vi "Do.vi"(8 "error in (no error)":errorcluster, 9 "Events":refnum<class "Events.lvclass">, 10 "Message Loop Data in":T1, 11 "IRegister in":refnum<class "IRegister.lvclass">) -> (0 "error out":errorcluster, 1 "Write request":T10, 2 "Message Loop Data out":T1, 3 "IRegister out":refnum<class "IRegister.lvclass">)   [LabVIEW 2020, in "wamplv.lvlib" / "IRegister.lvclass"]
uses:
  IRegister.lvclass
  WAMP Client/API/TypeDefs/WAMP error (JSON).ctl
  wamplv.lvlib
  WAMP Client/API/TypeDefs/Combined error.ctl
  WAMP Client/Private/TypeDef/Success or error (JSON).ctl
  WAMP Client/Private/TypeDef/Publish Requests Map.ctl
  WAMP Client/Private/TypeDef/Endpoint Data.ctl
  Call/ICallRequest/ICallRequest.lvclass
  WAMP Client/Private/TypeDef/CALL Request Map.ctl
  WAMP Client/Private/TypeDef/SUBSCRIBE Requests Map.ctl
  WAMP Client/Private/TypeDef/Subscriptions Map.ctl
  WAMP Client/Private/TypeDef/Unsubscribe Requests Map.ctl
  WAMP Client/Private/TypeDef/Unregister request (JSON).ctl
  WAMP Client/Private/TypeDef/Unregister requests map.ctl
  WAMP Client/Private/TypeDef/Message Loop Data.ctl
  TypeDefs/Transport type.ctl
  WAMP Client/Private/TypeDef/Write queue item.ctl
  Events/EventsParent/Events.lvclass
  Subscribe/ISubscribe/ISubscribe.lvclass
  Publish/IPublish/IPublish.lvclass
  Message loop classes/Subscription details/SubscriptionDetailsParent/SubscriptionDetailsParent.lvclass
  Unsubscribe/IUnsubscribe/IUnsubscribe.lvclass
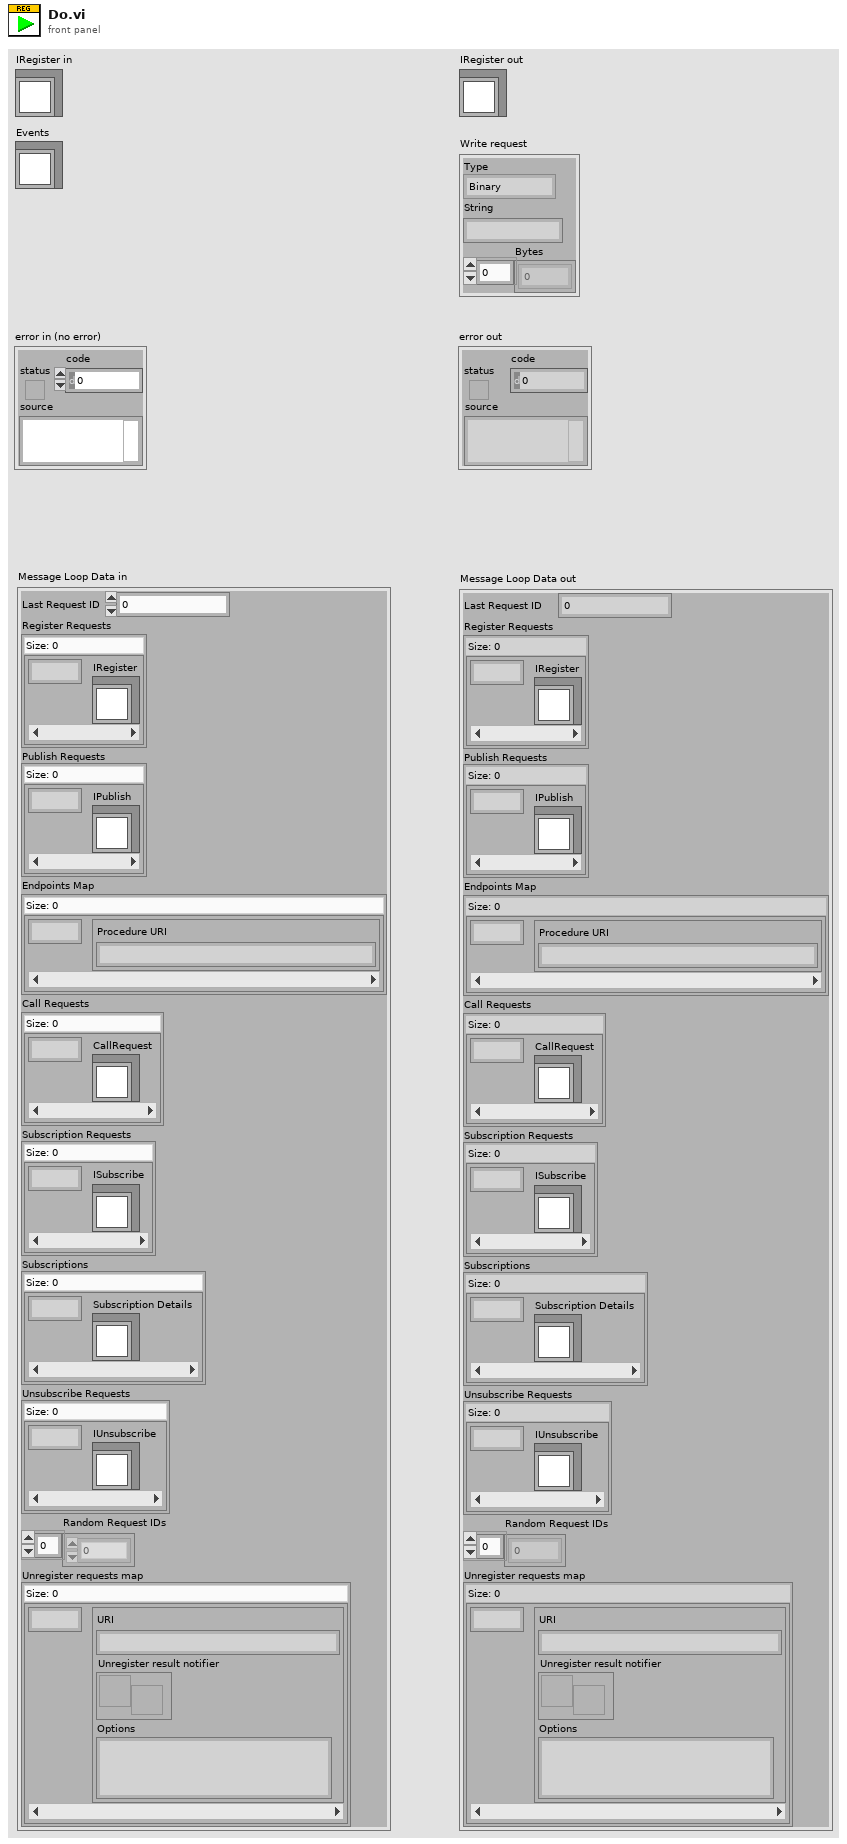
[diagram p1: front panel]
types:
  T1 = typedef "wamplv.lvlib/Message Loop Data.ctl" = cluster{"Last Request ID":u64, "Register Requests":map{u64, refnum<class "IRegister.lvclass">}, "Publish Requests":T2, "Endpoints Map":map{u64, T3}, "Call Requests":T4, "Subscription Requests":T5, "Subscriptions":T6, "Unsubscribe Requests":T7, "Random Request IDs":u64[], "Unregister requests map":T8}
  T2 = typedef "wamplv.lvlib/Publish Requests Map.ctl" = map{u64, refnum<class "IPublish.lvclass">}
  T3 = typedef "wamplv.lvlib/Endpoint Data.ctl" = cluster{"Procedure URI":string}
  T4 = typedef "wamplv.lvlib/CALL Request Map.ctl" = map{u64, refnum<class "ICallRequest.lvclass">}
  T5 = typedef "wamplv.lvlib/SUBSCRIBE Requests Map.ctl" = map{u64, refnum<class "ISubscribe.lvclass">}
  T6 = typedef "wamplv.lvlib/Subscriptions Map.ctl" = map{u64, refnum<class "SubscriptionDetailsParent.lvclass">}
  T7 = typedef "wamplv.lvlib/Unsubscribe Requests Map.ctl" = map{u64, refnum<class "IUnsubscribe.lvclass">}
  T8 = typedef "wamplv.lvlib/Unregister requests map.ctl" = map{u64, T9}
  T9 = typedef "wamplv.lvlib/Unregister request (JSON).ctl" = cluster{"URI":string, "Unregister result notifier":refnum<notifier>, "Options":string}
  T10 = typedef "wamplv.lvlib/Write queue item.ctl" = cluster{"Type":T11, "String":string, "Bytes":u8[]}
  T11 = typedef "wamplv.lvlib/Transport type.ctl" = enum16{"Binary", "Text"}
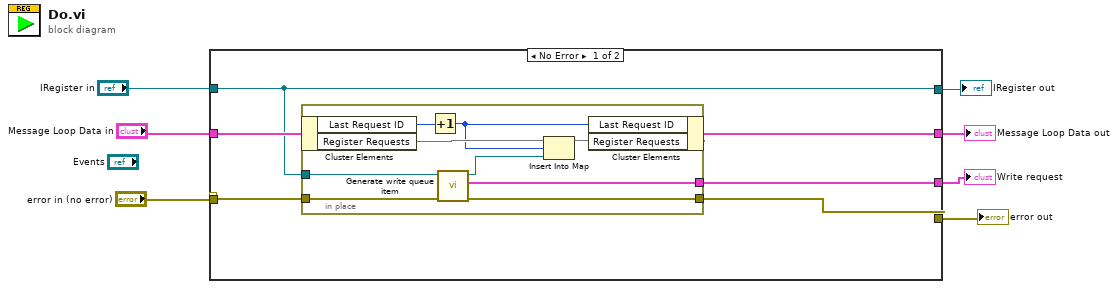
[diagram p0: block diagram]
diagram:
  n1 = case shown="No Error" {
    selector: _ -> [w10 w25]
    tunnel: [w9 w25] -> w5
    tunnel: "IRegister in" -> [w11 w23]
    tunnel: "Message Loop Data in" -> [w13 w24]
    tunnel: [w12 w24] -> w4
    tunnel: "error in (no error)" -> [_ _]
    tunnel: [w11 w23] -> w2
    tunnel: [w8 _] -> w1
    frame No Error {
      n2 = in-place {
        in-place-border: w11 -> [w17]
        in-place-border: w10 -> [w18]
        in-place-border: [w15] -> w9
        in-place-border: [w14] -> w8
        n3 = in-place-cluster #1(w13) -> ("Last Request ID"=w22:u64, "Register Requests"=w21:map{u64, refnum<class "IRegister.lvclass">})
        n4 = Increment(x=w22) -> (x+1=w20:u64)
        n5 = call-dynamic "Generate write queue item.vi"("error in (no error)"=w18, "IRegister in"=w17) -> ("error out"=w15:errorcluster, "Write queue item"=w14:T10, "IRegister out"=w16:refnum<class "IRegister.lvclass">)  [unwired: 7 in]
        n6 = Insert Into Map(map in=w21, key=w20, value=w16) -> (map out=w19:map{u64, refnum<class "IRegister.lvclass">})  [unwired: 2 out]
        n7 = in-place-cluster #1("Last Request ID"=w20, "Register Requests"=w19) -> (w12:T1)
      }
    }
    frame Error {
    }
  }
  "error out" <- w5
  "IRegister out" <- w2
  "Write request" <- w1
  "Message Loop Data out" <- w4
